vi "GetMCSAFFTByName.vi"(8 "error in (no error)":errorcluster, 10 "Channel Name":string, 11 "MCSA FFT in":T1) -> (0 "error out":errorcluster, 1 "MCSA FFT out":T1, 2 "Found?":bool)   [LabVIEW 2017, in "McsaUtilities.lvlib"]
uses:
  <vilib>/addons/InsightCM/Utilities/MCSA/McsaUtilities.lvlib
  <vilib>/addons/InsightCM/Utilities/Analysis/MCSA/controls/McsaFFT.ctl
  <vilib>/addons/InsightCM/Utilities/Analysis/MCSA/McsaAnalysisFunctions.lvlib
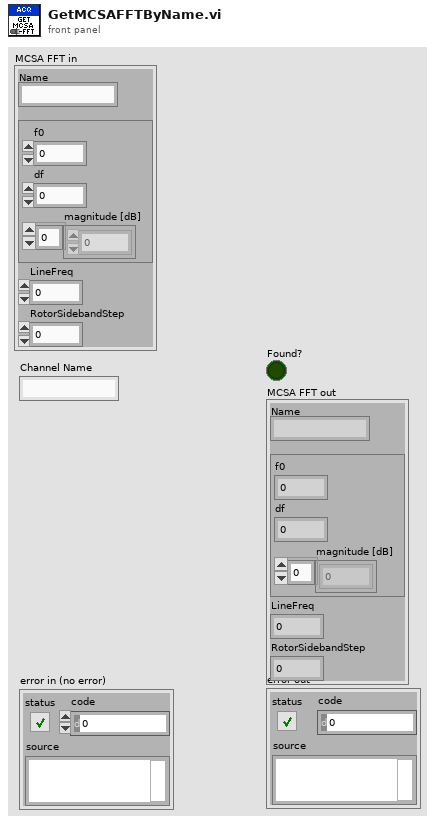
[diagram p1: front panel]
types:
  T1 = typedef "McsaAnalysisFunctions.lvlib/McsaFFT.ctl" = cluster{"Name":string, "Spectrum":cluster{"f0":dbl, "df":dbl, "magnitude [dB]":dbl[]}, "LineFreq":dbl, "RotorSidebandStep":dbl}
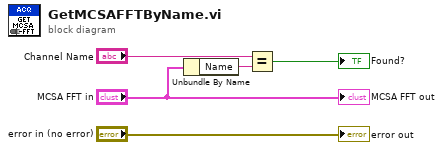
[diagram p0: block diagram]
diagram:
  n1 = Unbundle By Name("MCSA FFT in") -> ("Name"=w2:string)
  n2 = Equal?(x="Channel Name", y=w2) -> (x = y?=→"Found?":bool)
  "error out" <- "error in (no error)"
  "MCSA FFT out" <- "MCSA FFT in"
